vi "Write File.vi"(8 "error in (no error)":errorcluster, 11 "Data.TDMS in":refnum<class "Data.TDMS.lvclass">) -> (0 "error out":errorcluster, 3 "Data.TDMS out":refnum<class "Data.TDMS.lvclass">)   [LabVIEW 2016, in "Data.TDMS.lvclass"]
uses:
  Data.TDMS.lvclass
  Data/Data.lvclass
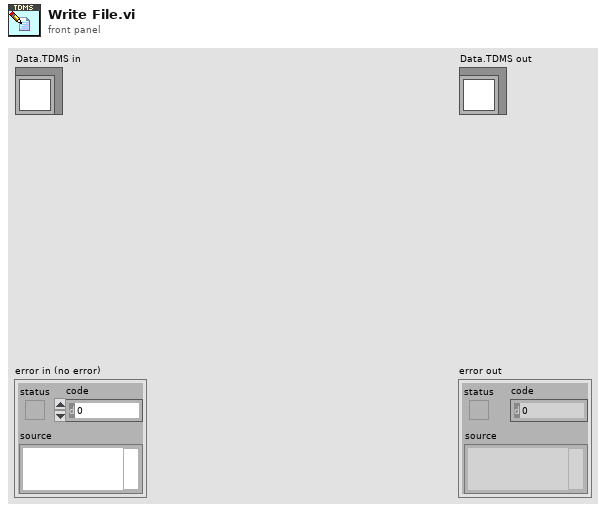
[diagram p1: front panel]
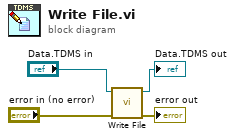
[diagram p0: block diagram]
diagram:
  n1 = call-parent "Write File.vi"("error in (no error)"="error in (no error)", "Data in"="Data.TDMS in") -> ("error out"=→"error out":errorcluster, "Data out"=→"Data.TDMS out":refnum<class "Data.TDMS.lvclass">)  [unwired: 8 in]
